vi "Discover DCM Dialog.vi"() -> (0 "Canceled?":bool, 3 "DCM Target Out":T1 caption="RIO Device", 5 "Path Out":path)   [LabVIEW 2016, in "DCM System Explorer.lvlib"]
uses:
  DCM System Explorer.lvlib
  <vilib>/userdefined/Silver/nirio_resource_slv.ctl
panel:
  in  "DCM Target":T1 caption="RIO Device"
  in  "Custom Bitfile Path (optional)":path
  in  "Cancel":bool
  in  "OK":bool
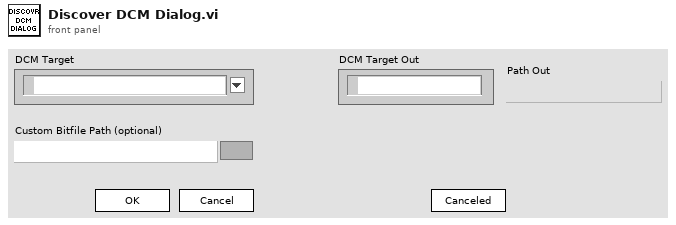
[diagram p1: front panel]
types:
  T1 = typedef "nirio_resource_slv.ctl" = tag
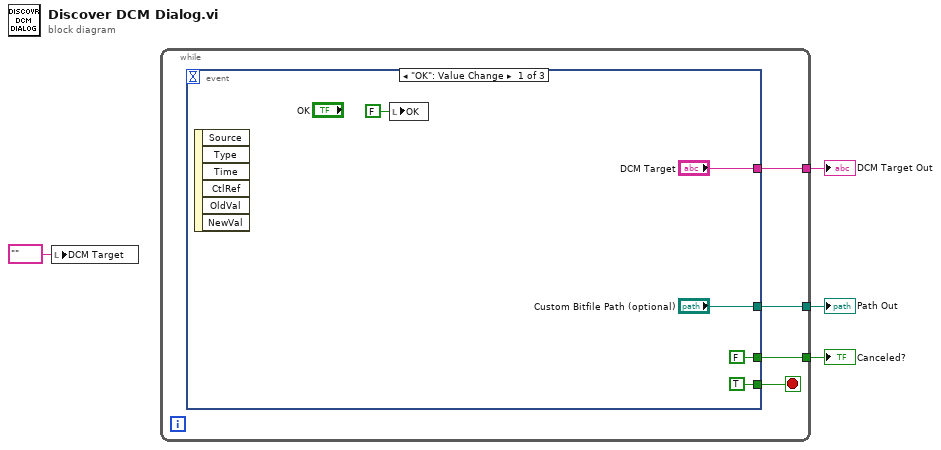
[diagram p0: block diagram]
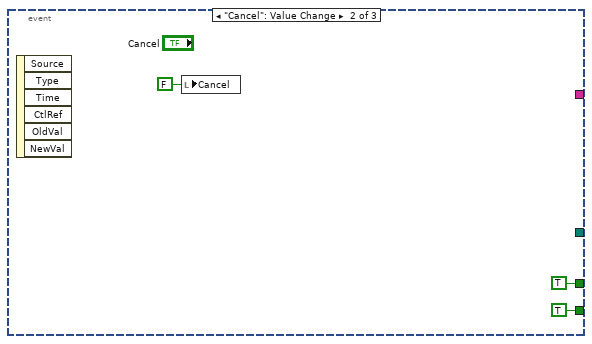
[diagram p2: hidden frame]
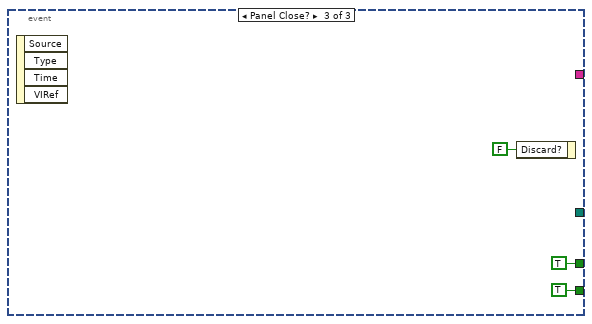
[diagram p3: hidden frame]
diagram:
  n1 = local write "DCM Target"(T1 "" ("DCM Target")) -> ()
  n2 = while {
    tunnel: [w8] -> w1
    tunnel: [w6] -> w4
    tunnel: [w5] -> w3
    stop <- w7 stop-if-true
    n3 = event shown="[0] \"OK\": Value Change" {
      selector: _ -> [_ _ _]
      dyn-events: _ -> [_ _ _]
      timeout: _ -> [_ _ _]
      tunnel: ["DCM Target" _ _] -> w8
      tunnel: [TRUE ("Discard?") TRUE ("Discard?") TRUE ("Discard?")] -> w7
      tunnel: [FALSE ("Value (Signaling)") TRUE ("Value (Signaling)") TRUE ("Value (Signaling)")] -> w6
      tunnel: ["Custom Bitfile Path (optional)" _ _] -> w5
      event "OK": Value Change {
        n4 = event-data() -> ()  [unwired: 1 in, 6 out]
        n5 = local write "OK"(FALSE ("OK")) -> ()
      }
      event "Cancel": Value Change {
        n6 = event-data() -> ()  [unwired: 1 in, 6 out]
        n7 = local write "Cancel"(FALSE ("Cancel")) -> ()
      }
      event Panel Close? {
        n8 = event-data() -> ()  [unwired: 1 in, 4 out]
        n9 = event-data("Discard?"=FALSE) -> ()  [unwired: 1 in, 1 out]
      }
    }
  }
  "Canceled?" <- w4
  "Path Out" <- w3
  "DCM Target Out" <- w1
